vi "Mode Code 17 with Start Stop and Status.vi"(7 "base name for channel aliases":string, 8 "error in":errorcluster, 11 "Loopback in":refnum<class "Loopback.lvclass">) -> (0 "error out":errorcluster, 3 "Loopback out":refnum<class "Loopback.lvclass">)   [LabVIEW 2020, in "Loopback.lvclass"]
uses:
  Loopback.lvclass
  niveristand-custom-device-testing-tools/VeriStandTestUtilities/VeriStandTestUtilities.lvlib
  <vilib>/numeric/Random Number (Range) U64.vi
  <vilib>/NI VeriStand/Execution/Workspace/NI_VS Workspace ExecutionAPI.lvlib
  <vilib>/NI VeriStand/Execution/Workspace/NI VeriStand - Set Single Channel Value.vi
  cdeade30-b699-48a0-a98c-dc2f8a2cbc9e.vi
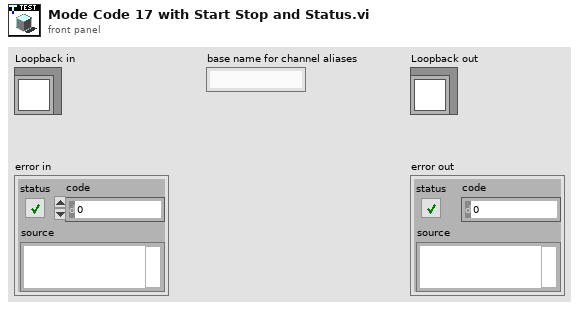
[diagram p1: front panel]
types:
  T1 = typedef "NI_VS Workspace ExecutionAPI.lvlib/WorkspaceAPI.ctl" = refnum<k24>
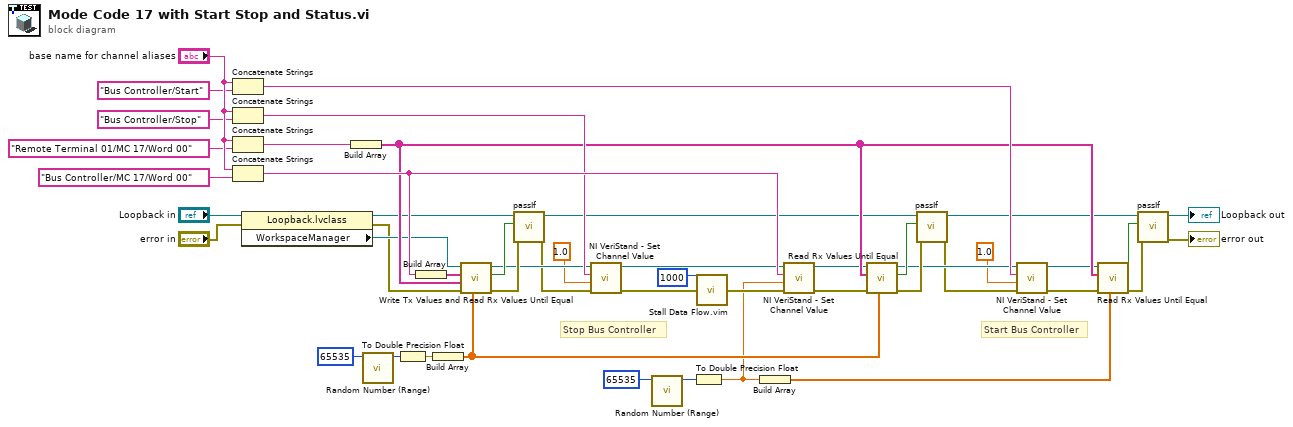
[diagram p0: block diagram]
diagram:
  # "Start Bus Controller"
  # "Stop Bus Controller"
  n1 = Concatenate Strings("base name for channel aliases", "Bus Controller/Start" ("Channel")) -> (w41:string)
  n2 = Concatenate Strings("base name for channel aliases", "Bus Controller/Stop" ("Channel")) -> (w43:string)
  n3 = Concatenate Strings("base name for channel aliases", "Remote Terminal 01/MC 17/Word 00" ("Channel")) -> (w45:string)
  n4 = Concatenate Strings("base name for channel aliases", "Bus Controller/MC 17/Word 00" ("Channel")) -> (w47:string)
  n5 = property class="Loopback.lvclass"(reference="Loopback in", error in="error in") -> (reference out=w1:refnum<class "Loopback.lvclass">, error out=w2:errorcluster, "WorkspaceManager"=w3:T1)
  n6 = Build Array(w45) -> (w37:string[])
  n7 = call-poly <vilib>:"Random Number (Range).vi"("upper bound (100)"=u64 65535) -> ("number"=w6:u64)  [unwired: 10 in]
  n8 = To Double Precision Float(number=w6) -> (double precision float=w21:dbl)
  n9 = Build Array(w47) -> (w22:string[])
  n10 = Build Array(w21) -> (w30:dbl[])
  n11 = call "Write Tx Values and Read Rx Values Until Equal.vi"("Tx values"=w30, "error in"=w2, "Rx aliases"=w37, "Tx aliases"=w22, "workspace manager in"=w3) -> ("error out"=w24:errorcluster, "values equal"=w25:bool, "workspace manager out"=w23:T1)  [unwired: 4 in]
  n12 = call-dynamic "passIf.vi"("error in (no error)"=w24, "pass"=w25, "TestCase in"=w1) -> ("error out"=w19:errorcluster, "TestCase out"=w20:refnum<class "Loopback.lvclass">)  [unwired: 7 in]
  n13 = call-poly <vilib>:"NI VeriStand - Set Channel Value.vi"("error in (no error)"=w19, "Value"=1.0, "Channel"=w43, "WorkspaceManager in"=w23) -> ("error out"=w17:errorcluster, "WorkspaceManager out"=w14:T1)  [unwired: 6 in]
  n14 = call-poly <vilib>:"Random Number (Range).vi"("upper bound (100)"=u64 65535) -> ("number"=w12:u64)  [unwired: 10 in]
  n15 = To Double Precision Float(number=w12) -> (double precision float=w8:dbl)
  n16 = call "Stall Data Flow.vim"("value in"=w17, "milliseconds to wait"=u32 1000) -> ("value out"=w15:errorcluster)  [unwired: 1 out]
  n17 = Build Array(w8) -> (w34:dbl[])
  n18 = call-poly <vilib>:"NI VeriStand - Set Channel Value.vi"("error in (no error)"=w15, "Value"=w8, "Channel"=w47, "WorkspaceManager in"=w14) -> ("error out"=w27:errorcluster, "WorkspaceManager out"=w26:T1)  [unwired: 6 in]
  n19 = call "Read Rx Values Until Equal.vi"("expected values"=w30, "error in"=w27, "Rx aliases"=w37, "workspace manager in"=w26) -> ("error out"=w29:errorcluster, "values equal expected"=w31:bool, "workspace manager out"=w28:T1)  [unwired: 5 in]
  n20 = call-dynamic "passIf.vi"("error in (no error)"=w29, "pass"=w31, "TestCase in"=w20) -> ("error out"=w10:errorcluster, "TestCase out"=w9:refnum<class "Loopback.lvclass">)  [unwired: 7 in]
  n21 = call-poly <vilib>:"NI VeriStand - Set Channel Value.vi"("error in (no error)"=w10, "Value"=1.0, "Channel"=w41, "WorkspaceManager in"=w28) -> ("error out"=w33:errorcluster, "WorkspaceManager out"=w32:T1)  [unwired: 6 in]
  n22 = call "Read Rx Values Until Equal.vi"("expected values"=w34, "error in"=w33, "Rx aliases"=w37, "workspace manager in"=w32) -> ("error out"=w35:errorcluster, "values equal expected"=w36:bool)  [unwired: 5 in, 1 out]
  n23 = call-dynamic "passIf.vi"("error in (no error)"=w35, "pass"=w36, "TestCase in"=w9) -> ("error out"=→"error out":errorcluster, "TestCase out"=→"Loopback out":refnum<class "Loopback.lvclass">)  [unwired: 7 in]
